vi "ReturnName.vi"(8 "error in (no error)":errorcluster, 11 "Interface in":refnum<class "Interface.lvclass">) -> (0 "error out":errorcluster, 2 "Name":string, 3 "Interface out":refnum<class "Interface.lvclass">)   [LabVIEW 2020, in "Mermaid.lvlib" / "Interface.lvclass"]
uses:
  Interface.lvclass
  Interface.lvclass/Interface.ctl
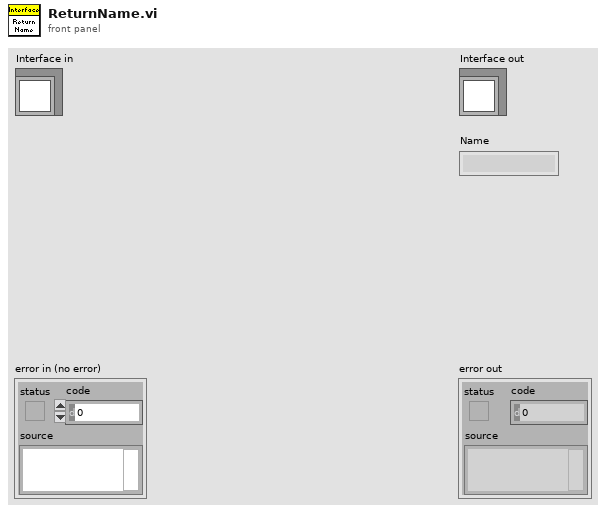
[diagram p1: front panel]
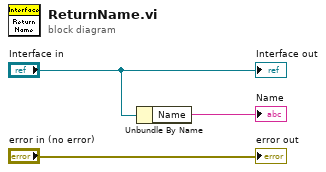
[diagram p0: block diagram]
diagram:
  n1 = Unbundle By Name("Interface in") -> ("Name"=→"Name":string)
  "error out" <- "error in (no error)"
  "Interface out" <- "Interface in"
